vi "GetDBPath.vi"(1 "Filename":string="PZJData.mdb") -> (0 "Connection":string="Provider=Microsoft.Jet.OLEDB.4.0;Data Source=C:\\Users\\jms\\Desktop\\MEMS WIN8\\MEMS WIN8\\Data Base\\PZJData.mdb;Persist Security Info=False")   [LabVIEW 2016]
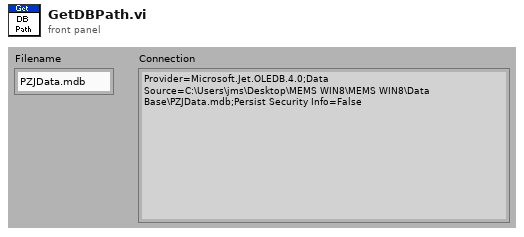
[diagram p1: front panel]
types:
  T1 = enum32{"invalid app kind", "Development System", "Run Time System", "Student Edition", "Embedded LabVIEW", "Evaluation", "Custom"}
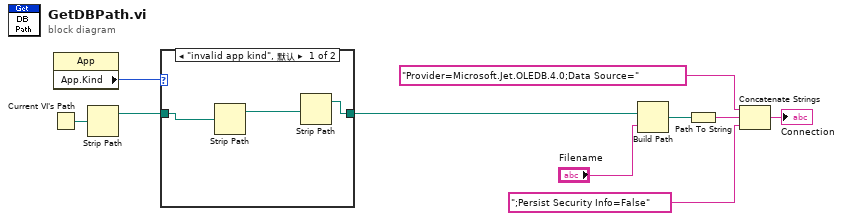
[diagram p0: block diagram]
diagram:
  n1 = Current VI's Path() -> (path=w4:path)
  n2 = property class="App"() -> ("App.Kind"=w3:T1)  [unwired: 2 in, 2 out]
  n3 = Strip Path(path=w4) -> (stripped path=w1:path)  [unwired: 1 out]
  n4 = case shown="\"invalid app kind\", 默认" w3 {
    tunnel: [w12 w14] -> w2
    tunnel: w1 -> [w13 w14]
    frame "invalid app kind", Default {
      n5 = Strip Path(path=w13) -> (stripped path=w11:path)  [unwired: 1 out]
      n6 = Strip Path(path=w11) -> (stripped path=w12:path)  [unwired: 1 out]
    }
    frame "Development System" {
    }
  }
  n7 = Build Path(base path=w2, name or relative path="Filename") -> (appended path=w9:path)
  n8 = Path To String(path=w9) -> (string=w8:string)
  n9 = Concatenate Strings("Provider=Microsoft.Jet.OLEDB.4.0;Data Source=" ("string"), w8, ";Persist Security Info=False" ("string")) -> (→"Connection":string)
